vi "Load EDS.vi"(8 "error in":errorcluster, 10 "EDS File Path":path, 11 "Interactor in":refnum<class "Interactor.lvclass">) -> (0 "error out":errorcluster, 3 "Interactor out":refnum<class "Interactor.lvclass">)   [LabVIEW 2024, in "Interactor.lvlib" / "Interactor.lvclass"]
uses:
  Interactor.lvclass
  Interactor.lvclass/Interactor.ctl
  Object Dictionary UI Messages/Populate OD Msg/Populate OD Msg.lvclass
  Home Messages/EDS File Loaded Msg/EDS File Loaded Msg.lvclass
  EDS-File-Viewer/Electronic Datasheet/Electronic Datasheet.lvclass
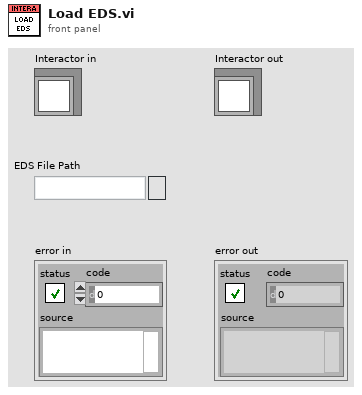
[diagram p1: front panel]
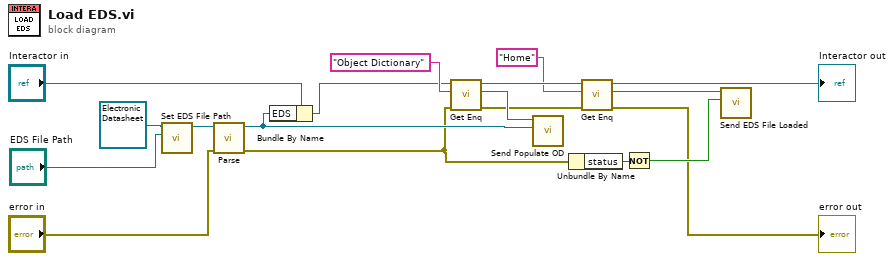
[diagram p0: block diagram]
diagram:
  n1 = call "Set EDS File Path.vi"("EDS File Path"="EDS File Path", "reference in"=refnum<class "Electronic Datasheet.lvclass"> refnum ("EDS in")) -> ("reference out"=w16:refnum<class "Electronic Datasheet.lvclass">)  [unwired: 8 in, 1 out]
  n2 = call "Parse.vi"("error in"="error in", "reference in"=w16) -> ("error out"=w4:errorcluster, "reference out"=w11:refnum<class "Electronic Datasheet.lvclass">)  [unwired: 8 in]
  n3 = Bundle By Name(cluster="Interactor in", "EDS"=w11) -> (w10:refnum<class "Interactor.lvclass">)
  n4 = call "Get Enq.vi"("error in"=w4, "Ident"="Object Dictionary", "Interactor in"=w10) -> ("error out"=w7:errorcluster, "Enq"=w13:refnum<class "Message Enqueuer.lvclass">, "Interactor out"=w18:refnum<class "Interactor.lvclass">)  [unwired: 6 in]
  n5 = call "Send Populate OD.vi"("EDS"=w11, "Message Enqueuer"=w13) -> ()  [unwired: 8 in, 2 out]
  n6 = Unbundle By Name(w4) -> ("status"=w3:bool)
  n7 = call "Get Enq.vi"("error in"=w7, "Ident"="Home", "Interactor in"=w18) -> ("error out"=→"error out":errorcluster, "Enq"=w5:refnum<class "Message Enqueuer.lvclass">, "Interactor out"=→"Interactor out":refnum<class "Interactor.lvclass">)  [unwired: 6 in]
  n8 = Not(x=w3) -> (.not. x?=w2:bool)
  n9 = call "Send EDS File Loaded.vi"("Valid?"=w2, "Message Enqueuer"=w5) -> ()  [unwired: 8 in, 2 out]
